vi "Multichannel Recording0.4.vi"() -> ()   [LabVIEW 2014]
uses:
  Enum State Typedef.ctl
  Consumer Data/ Consumer Event Com.ctl
  Data Producer States.ctl
  <vilib>/_DAQmxBase/Internals/DAQmxBase Read (Analog 2D DBL NChan NSamp).vi
  <vilib>/_DAQmxBase/Internals/DAQmxBase Create Channel (AI-Voltage-Basic).vi
  <vilib>/_DAQmxBase/Internals/DAQmxBase Timing (Sample Clock).vi
panel:
  out "Read Data":i32
  out "Data Producer State":T1=enum."Default"
  out "Data Consumer State":T2=enum."Default"
  in  "Open Button":bool
  in  "Tab Control":T3(tab)
  in  "Amplifier Channel 0":T4 {"Amplifier Model" items=["Select a Model", "AM 1700", "BMA 200"]}
  out "Channel 0 Chart":waveform(dbl)(graph)
  in  "User Data Channel 0":T5
  in  "Use Channel 0":bool caption="In Use?"
  out "Channel 1 Chart":waveform(dbl)(graph)
  in  "User Data Channel 1":T5
  in  "Amplifier Channel 1":T4 {"Amplifier Model" items=["Select a Model", "AM 1700", "BMA 200"]}
  in  "Use Channel 1":bool caption="In Use?"
  out "Channel 2 Chart":waveform(dbl)(graph)
  in  "User Data Channel 2":T5
  in  "Amplifier Channel 2":T4 {"Amplifier Model" items=["Select a Model", "AM 1700", "BMA 200"]}
  in  "Use Channel 2":bool caption="In Use?"
  out "Channel 3 Chart":waveform(dbl)(graph)
  in  "User Data Channel 3":T5
  in  "Amplifier Channel 3":T4 {"Amplifier Model" items=["Select a Model", "AM 1700", "BMA 200"]}
  in  "Use Channel 3":bool caption="In Use?"
  out "Overview Chart":waveform(dbl)[](graph)
  in  "Stop Preview":bool
  in  "OK Button":bool
  out "Event State":T6
  in  "Clear Display":bool
  in  "Preview Button":bool
  out "Iterations Recorded":i32
  in  "Recording Time (seconds)":dbl
  in  "Sample Rate":i32=1000
  in  "Stop Button":bool
  out "Start Time hr/min":string
  out "Date mm/dd/yy":string
  in  "Exit Button":bool
  in  "Record Button":bool
  # "MSU EFISH Lab Multi-Channel Electronic Pulse Recorder"
  # "Must enter numbers into here before you start"
  # "Blue for On\nOrange for Off"
  # "DC"
  # "AC"
  # "Blue for AC and Orange for DC"
  # "Blue for On\nOrange for Off"
  # "DC"
  # "AC"
  # "Blue for AC and Orange for DC"
  # "Blue for On\nOrange for Off"
  # "DC"
  # "AC"
  # "Blue for AC and Orange for DC"
  # "Blue for On\nOrange for Off"
  # "DC"
  # "AC"
  # "Blue for AC and Orange for DC"
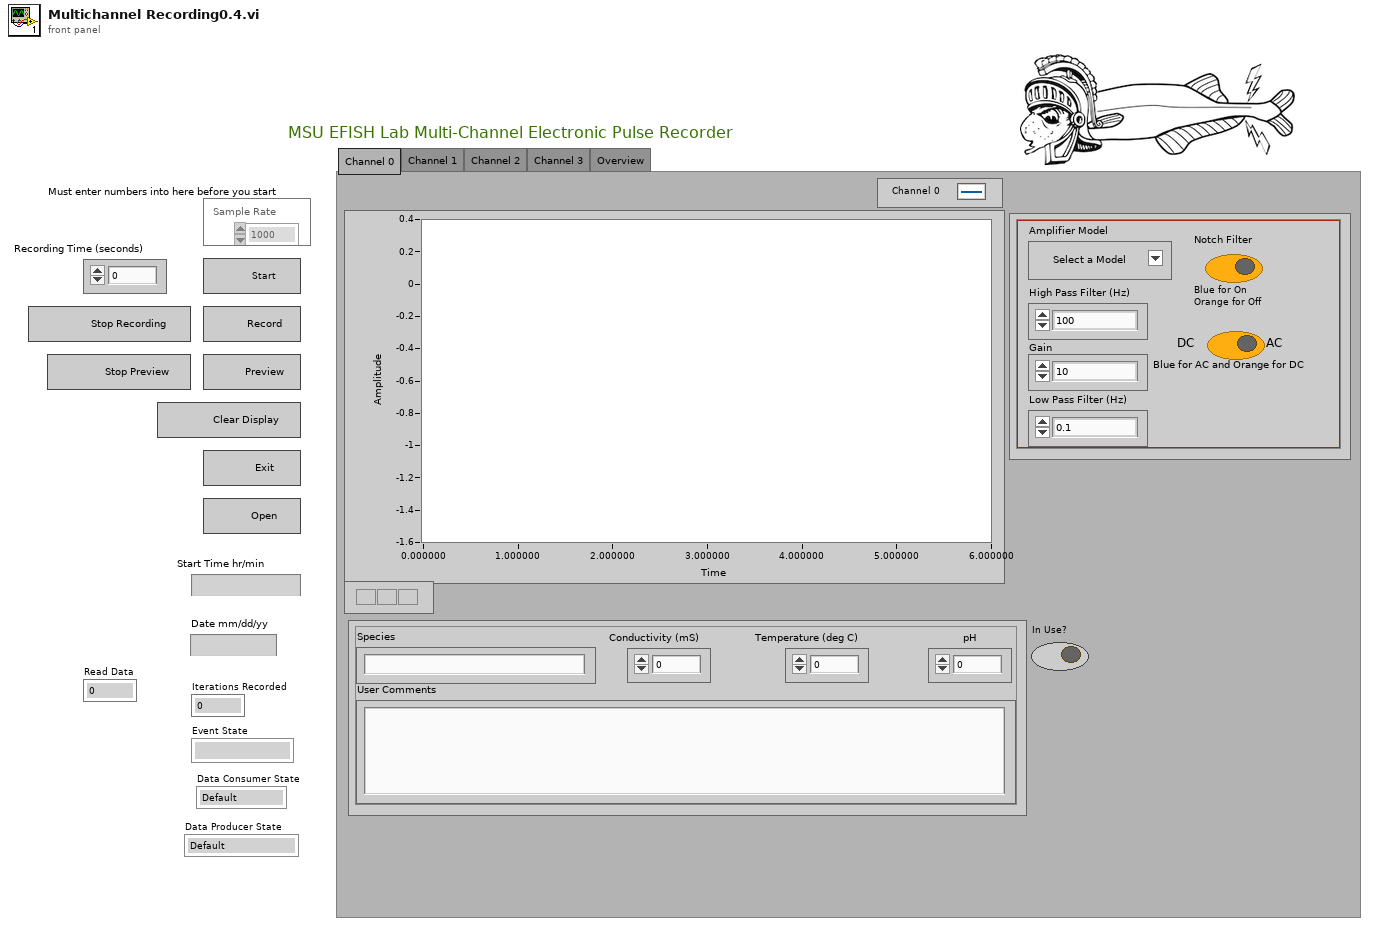
[diagram p1: front panel]
types:
  T1 = typedef "Data Producer States.ctl" = enum16{"Read Data", "Set Sample Clock", "Default", "Exit", "Preview"}
  T2 = typedef "Consumer Data/ Consumer Event Com.ctl" = enum16{"Recording", "Create File", "Clear Memory", "Default", "End File", "Exit", "Set Sample Clock", "Preview"}
  T3 = enum32{"Channel 0", "Channel 1", "Channel 2", "Channel 3", "Overview"}
  T4 = cluster{"Low Pass Filter (Hz)":enum16{"0.1", "1", "3", "10", "30", "100", "300"}, "Gain ":enum16{"10", "20", "50", "100", "200", "500", "1000", "2k", "5k", "10k", "20k", "50k"}, "High Pass Filter (Hz)":enum16{"100", "500", "1000", "3000", "5000", "10,000", "20,000", "30,000", "50,000"}, "Notch Filter":bool, "Amplifier Model":u16, "AC/DC Switch":bool}
  T5 = cluster{"pH":dbl, "Conductivity (mS)":dbl, "Temperature (deg C)":dbl, "User Comments":string, "Species":string}
  T6 = typedef "Enum State Typedef.ctl" = enum16{"", "Open FIle", "Beginning State", "Set the Sample Clock", "Prepreview Handling", "Clear Display", "Preview Data", "Stop", "Exit", "Record", "Create File"}
  T7 = enum8{"Enabled", "Disabled", "Disabled and Grayed Out"}
  T8 = enum16{"Recording", "Create File", "Clear Memory", "Default"}
  T9 = cluster{"Refnum out":refnum<k34>, "Refnum out":refnum<k34>, "Refnum out":refnum<k34>, "Refnum out":refnum<k34>}
  T10 = cluster{"Use Channel 0":bool, "Use Channel 1":bool, "Use Channel 2":bool, "Use Channel 3":bool}
  T11 = cluster{"tdms file out":refnum<k34>, "tdms file out":refnum<k34>, "tdms file out":refnum<k34>, "tdms file out":refnum<k34>}
  T12 = cluster{"Waveform":waveform(dbl), "Waveform":waveform(dbl), "Waveform":waveform(dbl), "Waveform":waveform(dbl)}
  T13 = cluster{"Waveform":waveform(dbl), "Waveform":waveform(dbl), "Waveform":waveform(dbl), "Waveform":waveform(dbl), waveform(dbl)[]}
  T14 = enum16{"Read Data", "Set Sample Clock", "Default", "Exit"}
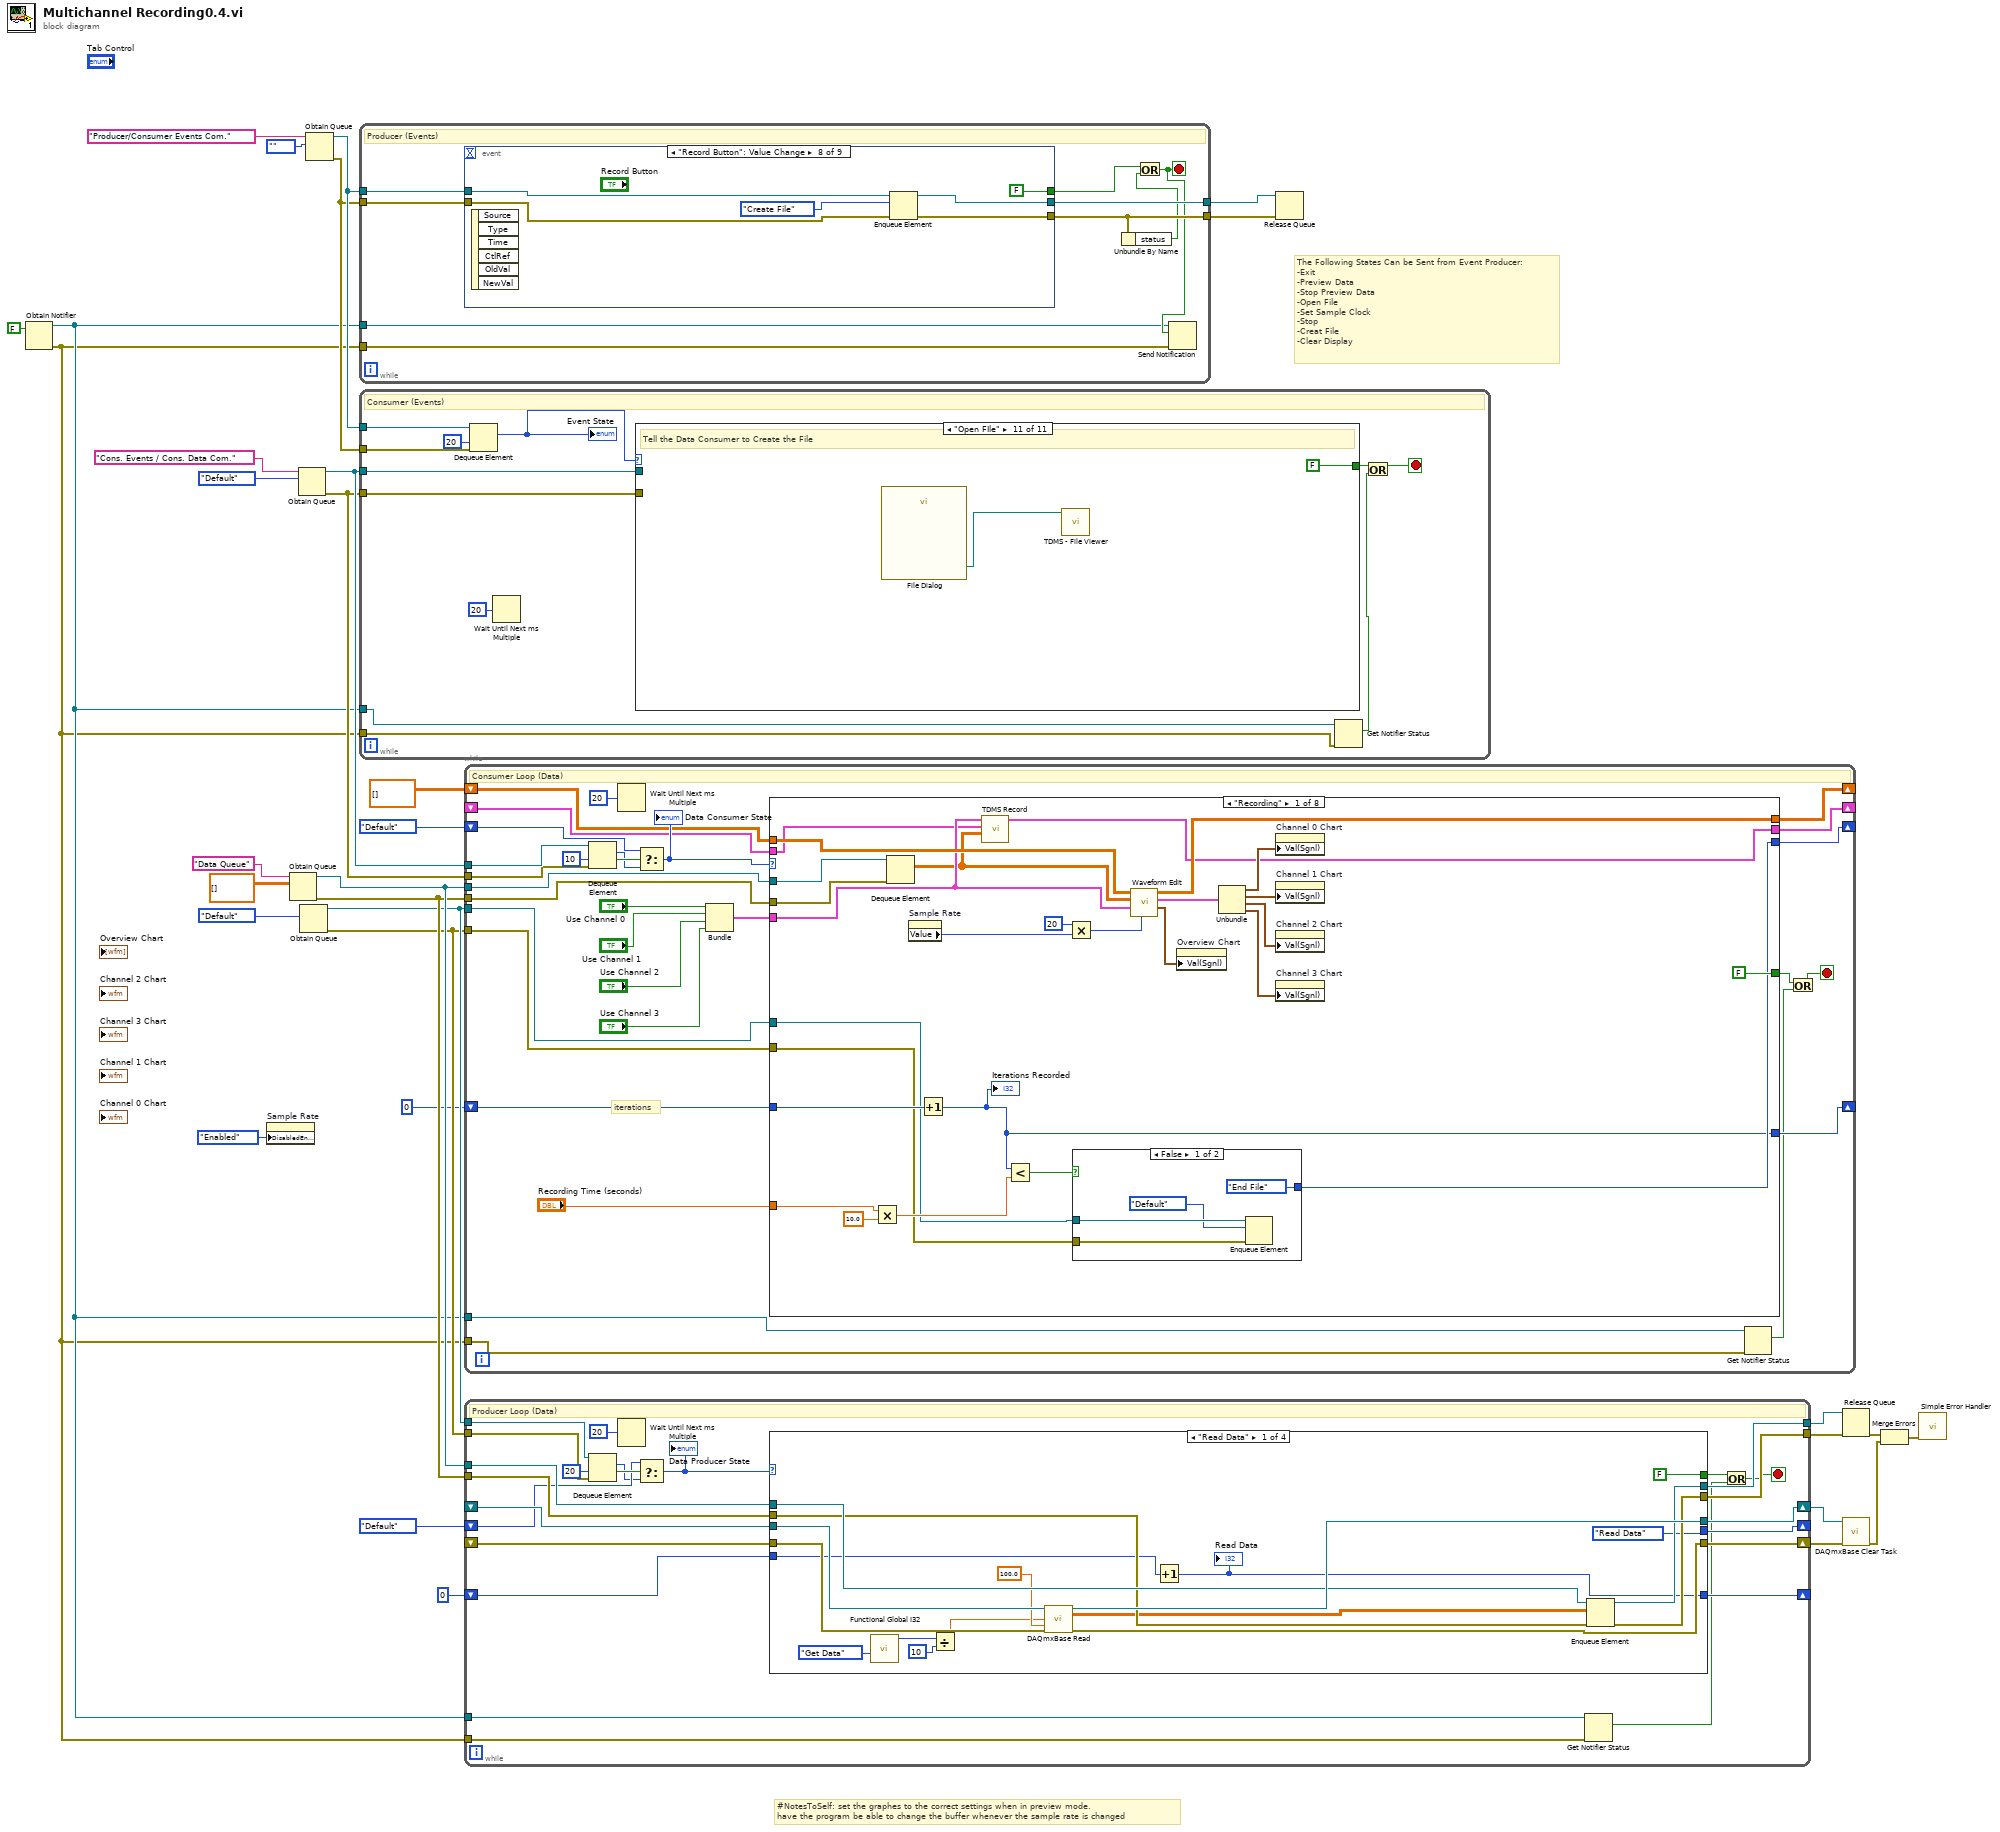
[diagram p0: block diagram]
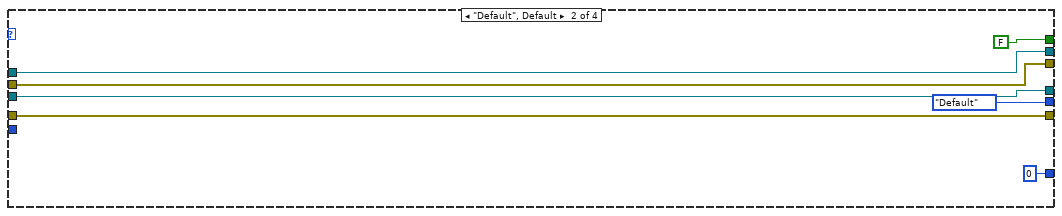
[diagram p2: hidden frame]
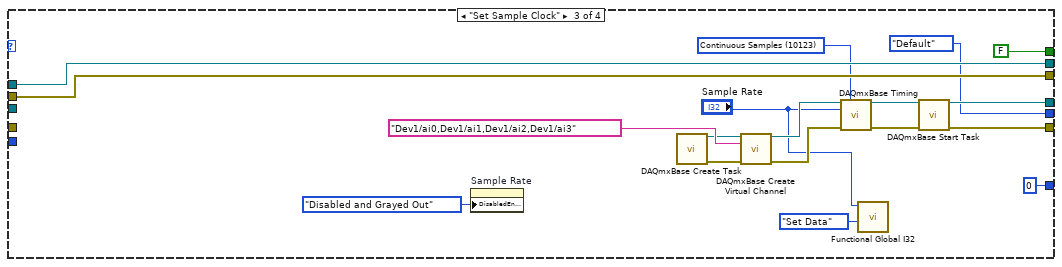
[diagram p3: hidden frame]
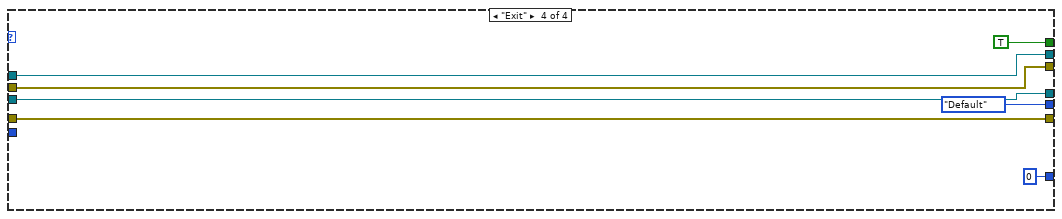
[diagram p4: hidden frame]
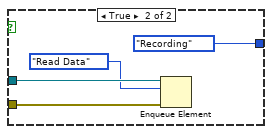
[diagram p5: hidden frame]
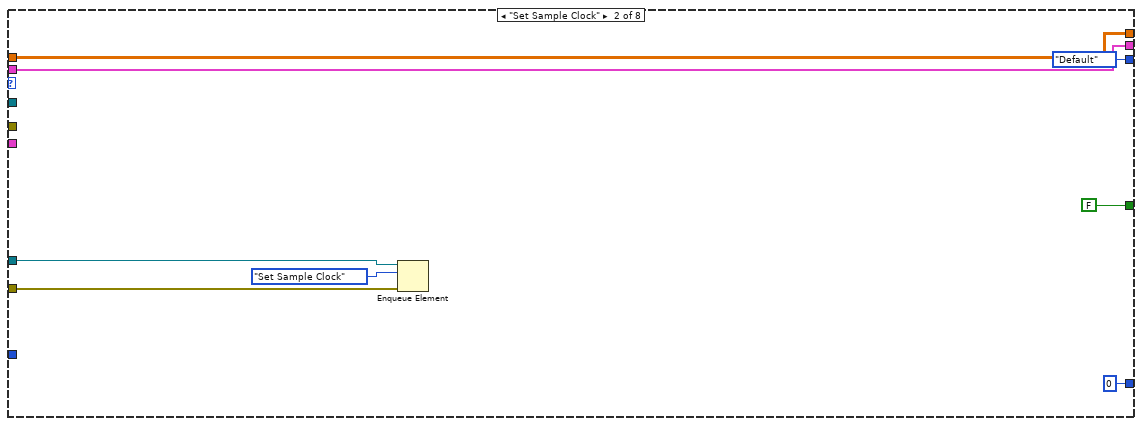
[diagram p6: hidden frame]
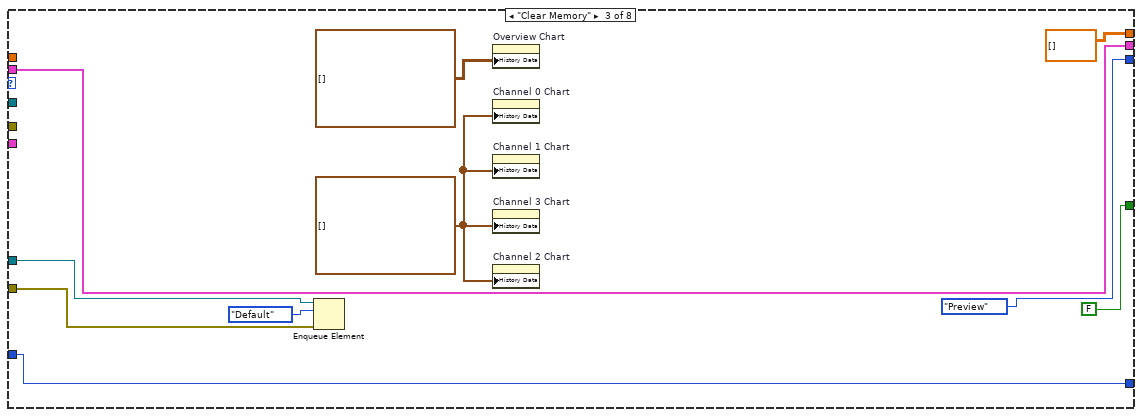
[diagram p7: hidden frame]
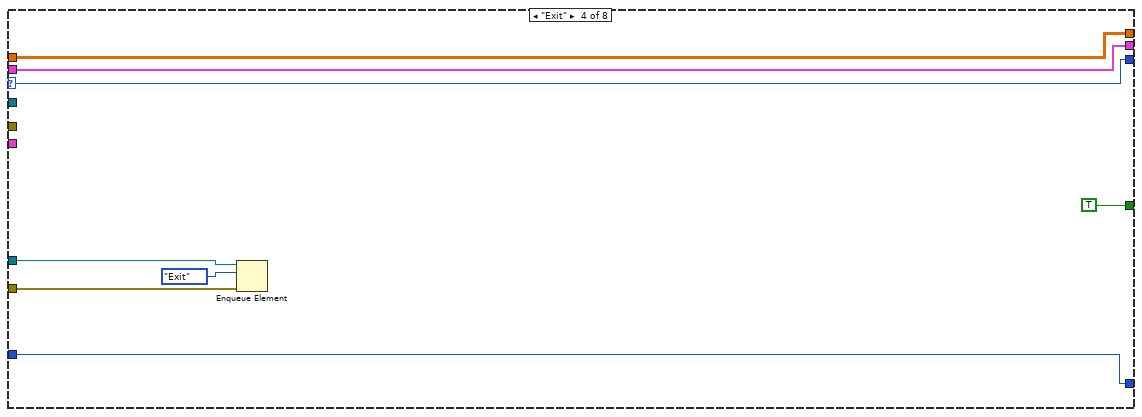
[diagram p8: hidden frame]
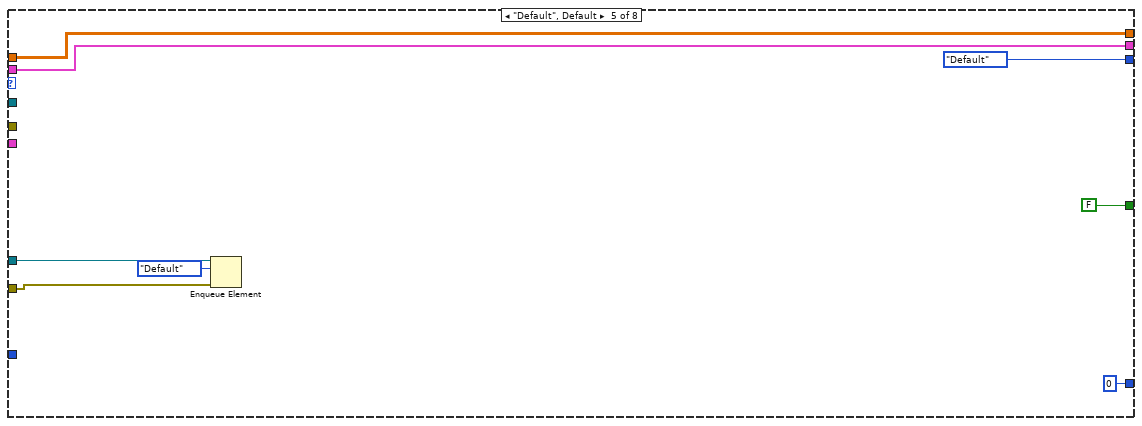
[diagram p9: hidden frame]
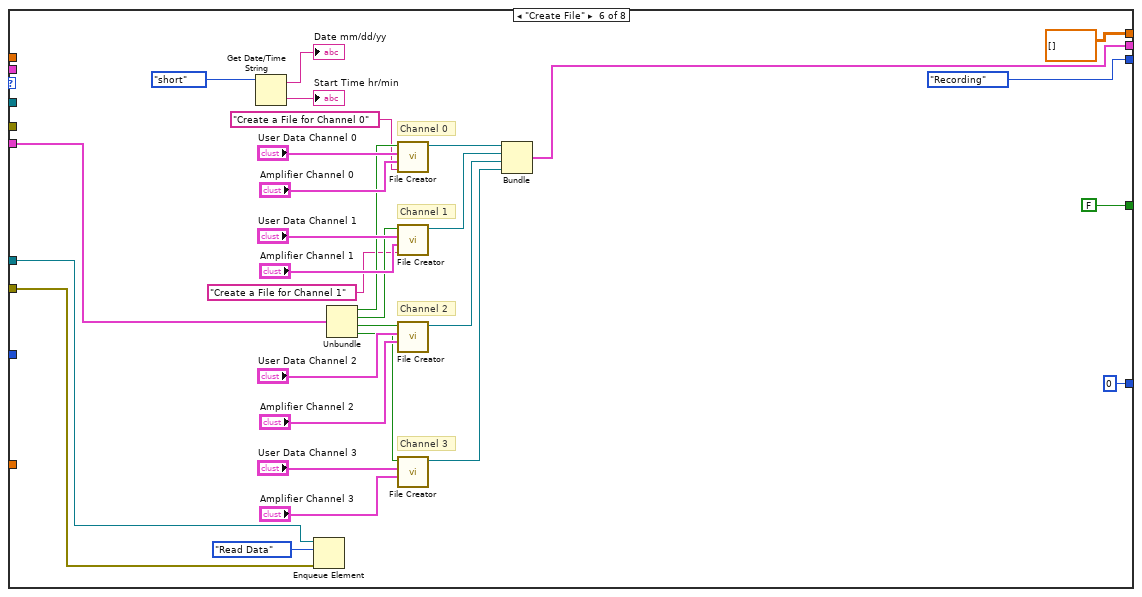
[diagram p10: hidden frame]
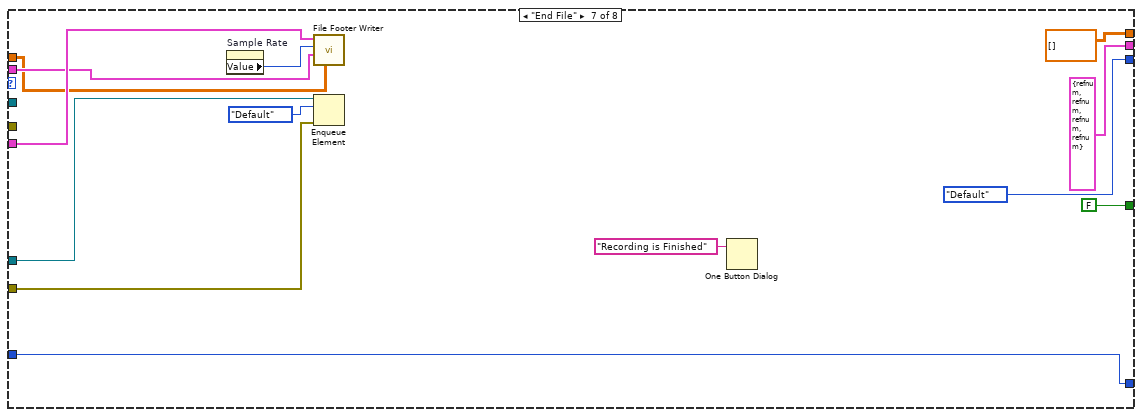
[diagram p11: hidden frame]
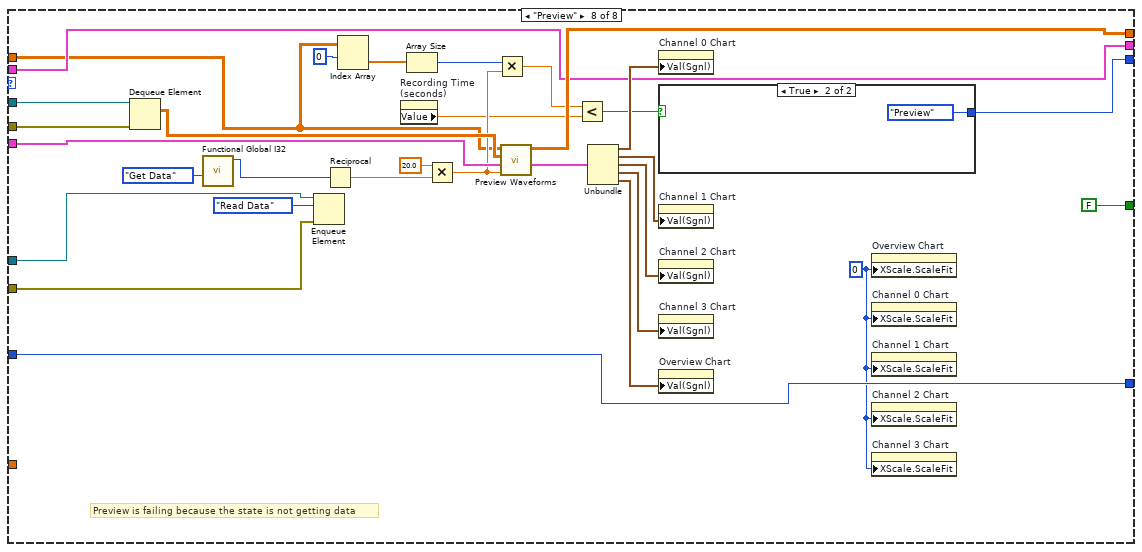
[diagram p12: hidden frame]
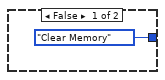
[diagram p13: hidden frame]
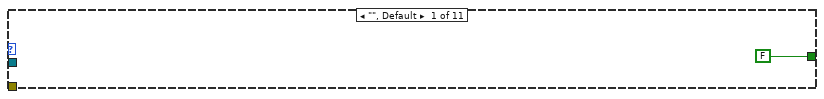
[diagram p14: hidden frame]
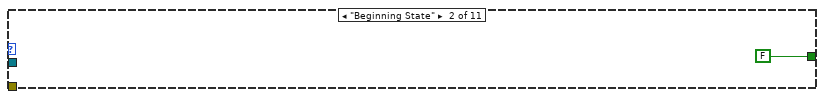
[diagram p15: hidden frame]
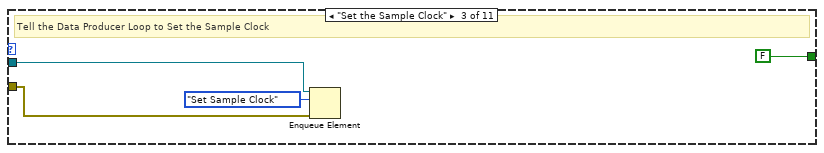
[diagram p16: hidden frame]
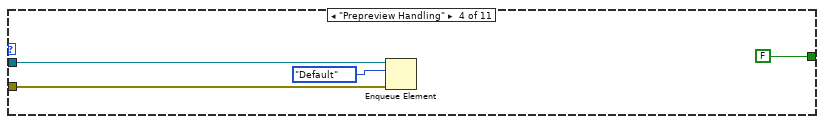
[diagram p17: hidden frame]
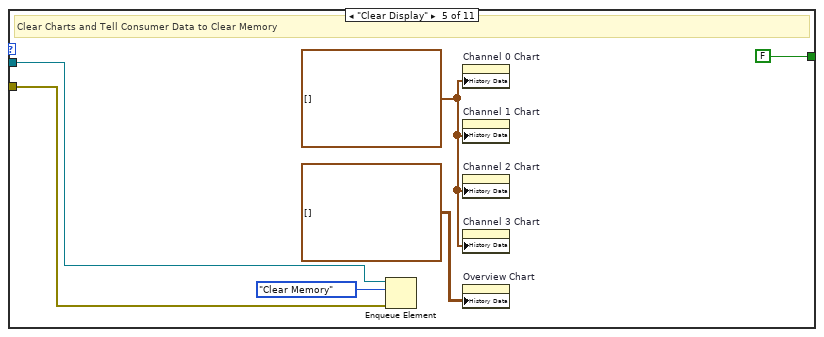
[diagram p18: hidden frame]
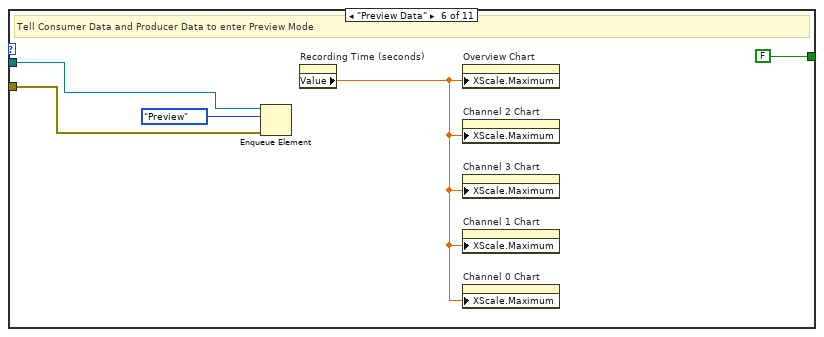
[diagram p19: hidden frame]
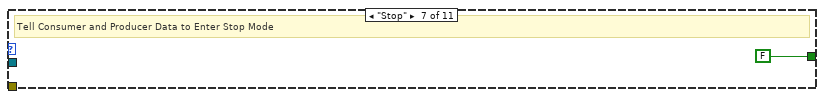
[diagram p20: hidden frame]
diagram:
  # "#NotesToSelf: set the graphes to the correct settings when in preview mode.\nhave the program be able to change the buffer whenever the sample rate is changed"
  # "The Following States Can be Sent from Event Producer:\n-Exit\n-Preview Data\n-Stop Preview Data\n-Open File\n-Set Sample Clock\n-Stop\n-Creat File\n-Clear Display"
  n1 = Obtain Notifier(notification data type=FALSE) -> (notifier out=w2:refnum<notifier>, error out=w1:errorcluster)  [unwired: 3 in, 1 out]
  n2 = property on="Sample Rate" class="DigNum (strict)"("DisabledEnum"=T7."Enabled" ("Disabled")) -> ()  [unwired: 2 in, 2 out]
  n3 = Obtain Queue(name (unnamed)="Data Queue", element data type=dbl[][] []) -> (queue out=w28:refnum<queue>, error out=w27:errorcluster)  [unwired: 3 in, 1 out]
  n4 = Obtain Queue(name (unnamed)="Cons. Events / Cons. Data Com.", element data type=Consumer_Data/_Consumer_Event_Com."Default") -> (queue out=w20:refnum<queue>, error out=w19:errorcluster)  [unwired: 3 in, 1 out]
  n5 = Obtain Queue(element data type=Data_Producer_States."Default") -> (queue out=w9:refnum<queue>, error out=w8:errorcluster)  [unwired: 4 in, 1 out]
  n6 = Obtain Queue(name (unnamed)="Producer/Consumer Events Com.", element data type=Enum_State_Typedef."" ("State")) -> (queue out=w32:refnum<queue>, error out=w31:errorcluster)  [unwired: 3 in, 1 out]
  n7 = while {
    tunnel: w32 -> [w42]
    tunnel: w31 -> [w41]
    tunnel: [w40] -> w26
    tunnel: [w39] -> w25
    tunnel: w2 -> [w35]
    tunnel: w1 -> [w34]
    stop <- w36 stop-if-true
    # "Producer (Events)"
    n8 = event shown="[7] \"Record Button\": Value Change" {
      selector: _ -> [_ _ _ _ _ _ _ _ _]
      dyn-events: _ -> [_ _ _ _ _ _ _ _ _]
      timeout: _ -> [_ _ _ _ _ _ _ _ _]
      tunnel: [FALSE ("Exit Button") "Exit Button" FALSE ("Exit Button") FALSE ("Exit Button") FALSE ("Exit Button") FALSE ("Exit Button") FALSE ("Exit Button") FALSE ("Exit Button") FALSE ("Exit Button")] -> w38
      tunnel: w42 -> [w44 w50 w57 w63 w69 w75 w81 w87 w93]
      tunnel: w41 -> [w43 w49 w56 w62 w68 w74 w80 w86 w92]
      tunnel: [w44 w47 w53 w59 w65 w71 w77 w83 w89] -> w40
      tunnel: [w43 w46 w52 w58 w64 w70 w76 w82 w88] -> w39
      event Timeout {
        n9 = event-data() -> ()  [unwired: 1 in, 3 out]
      }
      event "Exit Button": Value Change {
        n10 = event-data() -> ()  [unwired: 1 in, 1 out]
        n11 = Enqueue Element(queue=w50, element=Enum_State_Typedef."Exit", error in (no error)=w49) -> (queue out=w47:refnum<queue>, error out=w46:errorcluster)  [unwired: 1 in, 1 out]
      }
      event "Preview Button": Value Change {
        n12 = event-data() -> ()  [unwired: 1 in, 6 out]
        n13 = Enqueue Element(queue=w57, element=Enum_State_Typedef."Preview Data", error in (no error)=w56) -> (queue out=w53:refnum<queue>, error out=w52:errorcluster)  [unwired: 1 in, 1 out]
      }
      event "Stop Preview": Value Change {
        n14 = event-data() -> ()  [unwired: 1 in, 6 out]
        n15 = Enqueue Element(queue=w63, element=Enum_State_Typedef."Prepreview Handling", error in (no error)=w62) -> (queue out=w59:refnum<queue>, error out=w58:errorcluster)  [unwired: 1 in, 1 out]
      }
      event "Open Button": Value Change {
        n16 = event-data() -> ()  [unwired: 1 in, 6 out]
        n17 = Enqueue Element(queue=w69, element=Enum_State_Typedef."Open FIle", error in (no error)=w68) -> (queue out=w65:refnum<queue>, error out=w64:errorcluster)  [unwired: 1 in, 1 out]
      }
      event "OK Button": Value Change {
        n18 = event-data() -> ()  [unwired: 1 in, 6 out]
        n19 = Enqueue Element(queue=w75, element=Enum_State_Typedef."Set the Sample Clock", error in (no error)=w74) -> (queue out=w71:refnum<queue>, error out=w70:errorcluster)  [unwired: 1 in, 1 out]
      }
      event "Stop Button": Value Change {
        n20 = event-data() -> ()  [unwired: 1 in, 6 out]
        n21 = Enqueue Element(queue=w81, element=Enum_State_Typedef."Stop", error in (no error)=w80) -> (queue out=w77:refnum<queue>, error out=w76:errorcluster)  [unwired: 1 in, 1 out]
      }
      event "Record Button": Value Change {
        n22 = event-data() -> ()  [unwired: 1 in, 6 out]
        n23 = Enqueue Element(queue=w87, element=Enum_State_Typedef."Create File", error in (no error)=w86) -> (queue out=w83:refnum<queue>, error out=w82:errorcluster)  [unwired: 1 in, 1 out]
      }
      event "Clear Display": Value Change {
        n24 = event-data() -> ()  [unwired: 1 in, 6 out]
        n25 = Enqueue Element(queue=w93, element=Enum_State_Typedef."Clear Display", error in (no error)=w92) -> (queue out=w89:refnum<queue>, error out=w88:errorcluster)  [unwired: 1 in, 1 out]
      }
    }
    n26 = Unbundle By Name(w39) -> ("status"=w37:bool)
    n27 = Or(x=w38, y=w37) -> (x .or. y?=w36:bool)
    n28 = Send Notification(notification=w36, notifier=w35, error in (no error)=w34) -> ()  [unwired: 2 out]
  }
  n29 = while {
    tunnel: w32 -> [w105]
    tunnel: w31 -> [w104]
    tunnel: w20 -> [w103]
    tunnel: w19 -> [w102]
    tunnel: w2 -> [w97]
    tunnel: w1 -> [w96]
    stop <- w95 stop-if-true
    # "Consumer (Events)"
    n30 = Dequeue Element(queue=w105, timeout in ms (-1)=20, error in (no error)=w104) -> (element=w100:T6)  [unwired: 3 out]
    "Event State" <- w100
    n31 = Wait Until Next ms Multiple(millisecond multiple=u32 20) -> ()  [unwired: 1 out]
    n32 = case shown="\"Open FIle\"" w100 {
      tunnel: w103 -> [_ _ w110 w114 w118 w124 _ w131 _ w136 _]
      tunnel: w102 -> [_ _ w109 w113 w117 w123 _ w130 _ w135 _]
      tunnel: [FALSE FALSE FALSE FALSE FALSE FALSE FALSE TRUE FALSE FALSE FALSE] -> w101
      frame "", Default {
      }
      frame "Beginning State" {
      }
      frame "Set the Sample Clock" {
        # "Tell the Data Producer Loop to Set the Sample Clock"
        n33 = Enqueue Element(queue=w110, element=Consumer_Data/_Consumer_Event_Com."Set Sample Clock", error in (no error)=w109) -> ()  [unwired: 1 in, 3 out]
      }
      frame "Prepreview Handling" {
        n34 = Enqueue Element(queue=w114, element=Consumer_Data/_Consumer_Event_Com."Default", error in (no error)=w113) -> ()  [unwired: 1 in, 3 out]
      }
      frame "Clear Display" {
        w120 = waveform(dbl)[] [] ("History Data")
        # "Clear Charts and Tell Consumer Data to Clear Memory"
        n35 = Enqueue Element(queue=w118, element=Consumer_Data/_Consumer_Event_Com."Clear Memory", error in (no error)=w117) -> ()  [unwired: 1 in, 3 out]
        n36 = property on="Channel 0 Chart" class="WFChart (strict)"("History Data"=w120) -> ()  [unwired: 2 in, 2 out]
        n37 = property on="Channel 1 Chart" class="WFChart (strict)"("History Data"=w120) -> ()  [unwired: 2 in, 2 out]
        n38 = property on="Channel 2 Chart" class="WFChart (strict)"("History Data"=w120) -> ()  [unwired: 2 in, 2 out]
        n39 = property on="Channel 3 Chart" class="WFChart (strict)"("History Data"=w120) -> ()  [unwired: 2 in, 2 out]
        n40 = property on="Overview Chart" class="WFChart (strict)"("History Data"=waveform(dbl)[][] []) -> ()  [unwired: 2 in, 2 out]
      }
      frame "Preview Data" {
        # "Tell Consumer Data and Producer Data to enter Preview Mode"
        n41 = Enqueue Element(queue=w124, element=Consumer_Data/_Consumer_Event_Com."Preview", error in (no error)=w123) -> ()  [unwired: 1 in, 3 out]
        n42 = property on="Recording Time (seconds)" class="DigNum (strict)"() -> ("Value"=w125:dbl)  [unwired: 2 in, 2 out]
        n43 = property on="Overview Chart" class="WFChart (strict)"("XScale.Maximum"=w125) -> ()  [unwired: 2 in, 2 out]
        n44 = property on="Channel 2 Chart" class="WFChart (strict)"("XScale.Maximum"=w125) -> ()  [unwired: 2 in, 2 out]
        n45 = property on="Channel 3 Chart" class="WFChart (strict)"("XScale.Maximum"=w125) -> ()  [unwired: 2 in, 2 out]
        n46 = property on="Channel 1 Chart" class="WFChart (strict)"("XScale.Maximum"=w125) -> ()  [unwired: 2 in, 2 out]
        n47 = property on="Channel 0 Chart" class="WFChart (strict)"("XScale.Maximum"=w125) -> ()  [unwired: 2 in, 2 out]
      }
      frame "Stop" {
        # "Tell Consumer and Producer Data to Enter Stop Mode"
      }
      frame "Exit" {
        # "Tell Producer and Consumer Data to end themselves then End the Program"
        n48 = Enqueue Element(queue=w131, element=Consumer_Data/_Consumer_Event_Com."Exit", error in (no error)=w130) -> ()  [unwired: 1 in, 3 out]
      }
      frame "Record" {
        # "(I dont think that this case will exist)"
      }
      frame "Create File" {
        w133 = u8 2 ("X Scale.Scale Fit")
        # "Let Consumer Data Create File"
        n49 = Enqueue Element(queue=w136, element=Consumer_Data/_Consumer_Event_Com."Create File", error in (no error)=w135) -> ()  [unwired: 1 in, 3 out]
        n50 = property on="Overview Chart" class="WFChart (strict)"("XScale.ScaleFit"=w133) -> ()  [unwired: 2 in, 2 out]
        n51 = property on="Channel 3 Chart" class="WFChart (strict)"("XScale.ScaleFit"=w133) -> ()  [unwired: 2 in, 2 out]
        n52 = property on="Channel 2 Chart" class="WFChart (strict)"("XScale.ScaleFit"=w133) -> ()  [unwired: 2 in, 2 out]
        n53 = property on="Channel 1 Chart" class="WFChart (strict)"("XScale.ScaleFit"=w133) -> ()  [unwired: 2 in, 2 out]
        n54 = property on="Channel 0 Chart" class="WFChart (strict)"("XScale.ScaleFit"=w133) -> ()  [unwired: 2 in, 2 out]
      }
      frame "Open FIle" {
        # "Tell the Data Consumer to Create the File"
        n55 = call "File Dialog"() -> ("selected path"=w138:path)  [unwired: 12 in, 3 out]
        n56 = call <vilib>:"TDMS - File Viewer.vi"("file path"=w138) -> ()  [unwired: 5 in, 2 out]
      }
    }
    n57 = Get Notifier Status(notifier=w97, error in (no error)=w96) -> (current notification=w94:bool)  [unwired: 4 out]
    n58 = Or(x=w101, y=w94) -> (x .or. y?=w95:bool)
  }
  n59 = while {
    tunnel: w28 -> [w162]
    tunnel: w27 -> [w161]
    tunnel: w20 -> [w169]
    tunnel: w19 -> [w168]
    shift-right: [w163] -> _
    shift-left: Consumer_Data/_Consumer_Event_Com."Default" -> [w164]
    shift-right: [w157] -> _
    shift-left: dbl[][] [] -> [w160]
    shift-right: [w156] -> _
    shift-left: _ -> [w155]
    tunnel: w9 -> [w153]
    tunnel: w8 -> [w152]
    shift-right: [w148] -> _
    shift-left: 0 -> [w150]
    tunnel: w2 -> [w142]
    tunnel: w1 -> [w141]
    stop <- w144 stop-if-true
    # "iterations"
    # "Consumer Loop (Data)"
    n60 = Dequeue Element(queue=w169, timeout in ms (-1)=10, error in (no error)=w168) -> (element=w166:T2, timed out?=w167:bool)  [unwired: 2 out]
    n61 = Wait Until Next ms Multiple(millisecond multiple=u32 20) -> ()  [unwired: 1 out]
    n62 = Select(t=w164, s=w167, f=w166) -> (s? t:f=w165:T2)
    "Data Consumer State" <- w165
    n63 = Bundle("Use Channel 0"="Use Channel 0", "Use Channel 1"="Use Channel 1", "Use Channel 2"="Use Channel 2", "Use Channel 3"="Use Channel 3") -> (w158:T10)  [unwired: 1 in]
    n64 = case shown="\"Recording\"" w165 {
      selector: w165 -> [_ _ _ w228 _ _ _ _]
      tunnel: [w174 Consumer_Data/_Consumer_Event_Com."Default" Consumer_Data/_Consumer_Event_Com."Preview" w228 T8."Default" Consumer_Data/_Consumer_Event_Com."Recording" Consumer_Data/_Consumer_Event_Com."Default" w290] -> w163
      tunnel: w162 -> [w195 _ _ _ _ _ _ w312]
      tunnel: w161 -> [w194 _ _ _ _ _ _ w311]
      tunnel: [FALSE FALSE FALSE TRUE FALSE FALSE FALSE FALSE] -> w143
      tunnel: w160 -> [w193 w209 _ w229 w236 _ w279 w297]
      tunnel: w158 -> [w182 _ _ _ _ w262 w281 w309]
      tunnel: [w183 w209 dbl[][] [] ("Output Decimated Data") w229 w236 dbl[][] [] ("Output Decimated Data") dbl[][] [] ("Output Data") w306] -> w157
      tunnel: [w180 w208 w219 w227 w235 w245 T9 {"Refnum out"=refnum, "Refnum out"=refnum, "Refnum out"=refnum, "Refnum out"=refnum} ("Output TDMS File Cluster") w299] -> w156
      tunnel: w155 -> [w170 w208 w219 w227 w235 _ w280 w299]
      tunnel: w153 -> [w173 w212 w216 w226 w233 w244 w273 w288]
      tunnel: w152 -> [w172 w211 w215 w225 w232 w243 w272 w287]
      tunnel: w150 -> [w179 _ w213 w223 _ _ w270 w285]
      tunnel: "Recording Time (seconds)" -> [w178 _ _ _ _ _ _ _]
      tunnel: [w171 0 w213 w223 0 0 w270 w285] -> w148
      frame "Recording" {
        n65 = Multiply(x=w178, y=10.0) -> (x*y=w176:dbl)
        n66 = Dequeue Element(queue=w195, error in (no error)=w194) -> (element=w181:dbl[][])  [unwired: 1 in, 3 out]
        n67 = property on="Sample Rate" class="DigNum (strict)"() -> ("Value"=w192:i32)  [unwired: 2 in, 2 out]
        n68 = Increment(x=w179) -> (x+1=w171:i32)
        "Iterations Recorded" <- w171
        n69 = call "TDMS Record.vi"("Data"=w181, "Input TDMS File Cluster"=w170, "In Use Cluster"=w182) -> ("Output TDMS File Cluster"=w180:T11)  [unwired: 8 in]
        n70 = Less?(x=w171, y=w176) -> (x < y?=w175:bool)
        n71 = Multiply(x=20, y=w192) -> (x*y=w190:i32)
        n72 = case shown="False" w175 {
          tunnel: [Consumer_Data/_Consumer_Event_Com."End File" Consumer_Data/_Consumer_Event_Com."Recording"] -> w174
          tunnel: w173 -> [w199 w203]
          tunnel: w172 -> [w198 w202]
          frame False {
            n73 = Enqueue Element(queue=w199, element=Data_Producer_States."Default", error in (no error)=w198) -> ()  [unwired: 1 in, 3 out]
          }
          frame True {
            n74 = Enqueue Element(queue=w203, element=Data_Producer_States."Read Data", error in (no error)=w202) -> ()  [unwired: 1 in, 3 out]
          }
        }
        n75 = call "Waveform Edit.vi"("Change in Time"=w190, "In Use Cluster"=w182, "New Data"=w181, "Old Data"=w193) -> ("Overview Chart Data"=w184:waveform(dbl)[], "Output Waveform Cluster"=w189:T12, "Output Decimated Data"=w183:dbl[][])  [unwired: 5 in]
        n76 = property on="Overview Chart" class="WFChart (strict)"("Val(Sgnl)"=w184) -> ()  [unwired: 2 in, 2 out]
        n77 = Unbundle(w189) -> ("Waveform"=w188:waveform(dbl), "Waveform"=w187:waveform(dbl), "Waveform"=w186:waveform(dbl), "Waveform"=w185:waveform(dbl))
        n78 = property on="Channel 0 Chart" class="WFChart (strict)"("Val(Sgnl)"=w188) -> ()  [unwired: 2 in, 2 out]
        n79 = property on="Channel 1 Chart" class="WFChart (strict)"("Val(Sgnl)"=w187) -> ()  [unwired: 2 in, 2 out]
        n80 = property on="Channel 2 Chart" class="WFChart (strict)"("Val(Sgnl)"=w186) -> ()  [unwired: 2 in, 2 out]
        n81 = property on="Channel 3 Chart" class="WFChart (strict)"("Val(Sgnl)"=w185) -> ()  [unwired: 2 in, 2 out]
      }
      frame "Set Sample Clock" {
        n82 = Enqueue Element(queue=w212, element=Data_Producer_States."Set Sample Clock", error in (no error)=w211) -> ()  [unwired: 1 in, 3 out]
      }
      frame "Clear Memory" {
        w217 = waveform(dbl)[] [] ("History Data")
        n83 = Enqueue Element(queue=w216, element=Data_Producer_States."Default", error in (no error)=w215) -> ()  [unwired: 1 in, 3 out]
        n84 = property on="Overview Chart" class="WFChart (strict)"("History Data"=waveform(dbl)[][] []) -> ()  [unwired: 2 in, 2 out]
        n85 = property on="Channel 0 Chart" class="WFChart (strict)"("History Data"=w217) -> ()  [unwired: 2 in, 2 out]
        n86 = property on="Channel 1 Chart" class="WFChart (strict)"("History Data"=w217) -> ()  [unwired: 2 in, 2 out]
        n87 = property on="Channel 3 Chart" class="WFChart (strict)"("History Data"=w217) -> ()  [unwired: 2 in, 2 out]
        n88 = property on="Channel 2 Chart" class="WFChart (strict)"("History Data"=w217) -> ()  [unwired: 2 in, 2 out]
      }
      frame "Exit" {
        n89 = Enqueue Element(queue=w226, element=Data_Producer_States."Exit", error in (no error)=w225) -> ()  [unwired: 1 in, 3 out]
      }
      frame "Default", Default {
        n90 = Enqueue Element(queue=w233, element=Data_Producer_States."Default", error in (no error)=w232) -> ()  [unwired: 1 in, 3 out]
      }
      frame "Create File" {
        # "Channel 3"
        # "Channel 2"
        # "Channel 1"
        # "Channel 0"
        n91 = Get Date/Time String(date format (0)=enum16{"short", "long", "abbreviated"}."short") -> (date string=→"Date mm/dd/yy":string, time string=→"Start Time hr/min":string)  [unwired: 2 in]
        n92 = Enqueue Element(queue=w244, element=Data_Producer_States."Read Data", error in (no error)=w243) -> ()  [unwired: 1 in, 3 out]
        n93 = Unbundle(w262) -> ("Use Channel 0"=w255:bool, "Use Channel 1"=w254:bool, "Use Channel 2"=w253:bool, "Use Channel 3"=w252:bool)
        n94 = call "File Creator.vi"("prompt"="Create a File for Channel 0", "Amplifier Channel 1"="Amplifier Channel 0", "User Data Channel 1"="User Data Channel 0", "Use Channel in"=w255) -> ("Refnum out"=w251:refnum<k34>)  [unwired: 7 in]
        n95 = call "File Creator.vi"("prompt"="Create a File for Channel 1", "Amplifier Channel 1"="Amplifier Channel 1", "User Data Channel 1"="User Data Channel 1", "Use Channel in"=w254) -> ("Refnum out"=w250:refnum<k34>)  [unwired: 7 in]
        n96 = call "File Creator.vi"("Amplifier Channel 1"="Amplifier Channel 2", "User Data Channel 1"="User Data Channel 2", "Use Channel in"=w253) -> ("Refnum out"=w249:refnum<k34>)  [unwired: 8 in]
        n97 = call "File Creator.vi"("Amplifier Channel 1"="Amplifier Channel 3", "User Data Channel 1"="User Data Channel 3", "Use Channel in"=w252) -> ("Refnum out"=w248:refnum<k34>)  [unwired: 8 in]
        n98 = Bundle("Refnum out"=w251, "Refnum out"=w250, "Refnum out"=w249, "Refnum out"=w248) -> (w245:T9)  [unwired: 1 in]
      }
      frame "End File" {
        n99 = property on="Sample Rate" class="DigNum (strict)"() -> ("Value"=w278:i32)  [unwired: 2 in, 2 out]
        n100 = call "File Footer Writer.vi"("Old Data"=w279, "TDMS File Cluster"=w280, "Sample Rate"=w278, "In Use Cluster"=w281) -> ()  [unwired: 8 in]
        n101 = Enqueue Element(queue=w273, element=Data_Producer_States."Default", error in (no error)=w272) -> ()  [unwired: 1 in, 3 out]
        n102 = One Button Dialog(message="Recording is Finished") -> ()  [unwired: 1 in, 1 out]
      }
      frame "Preview" {
        w282 = u8 0 ("X Scale.Scale Fit")
        # "Preview is failing because the state is not getting data"
        n103 = Dequeue Element(queue=w312, error in (no error)=w311) -> (element=w310:dbl[][])  [unwired: 1 in, 3 out]
        n104 = call "Functional Global I32.vi"("Enum"=enum16{"Set Data", "Get Data"}."Get Data") -> ("Integer"=w283:i32)  [unwired: 10 in]
        n105 = Enqueue Element(queue=w288, element=Data_Producer_States."Read Data", error in (no error)=w287) -> ()  [unwired: 1 in, 3 out]
        n106 = Reciprocal(x=w283) -> (1/x=w308:dbl)
        n107 = Index Array(array=w297, index (row)=0) -> (element=w295:dbl[])  [unwired: 1 in]
        n108 = property on="Recording Time (seconds)" class="DigNum (strict)"() -> ("Value"=w292:dbl)  [unwired: 2 in, 2 out]
        n109 = Array Size(array=w295) -> (size(s)=w294:i32)
        n110 = Multiply(x=20.0, y=w308) -> (x*y=w298:dbl)
        n111 = Multiply(x=w294, y=w298) -> (x*y=w293:dbl)
        n112 = call "Preview Waveforms.vi"("Change in Time"=w298, "In Use Cluster"=w309, "Input Read Data"=w310, "Input Decimated Data"=w297) -> ("Output Waveform Cluster"=w305:T13, "Output Data"=w306:dbl[][])  [unwired: 6 in]
        n113 = Less?(x=w293, y=w292) -> (x < y?=w291:bool)
        n114 = Unbundle(w305) -> ("Waveform"=w304:waveform(dbl), "Waveform"=w303:waveform(dbl), "Waveform"=w302:waveform(dbl), "Waveform"=w301:waveform(dbl), w300:waveform(dbl)[])
        n115 = property on="Channel 0 Chart" class="WFChart (strict)"("Val(Sgnl)"=w304) -> ()  [unwired: 2 in, 2 out]
        n116 = case shown="True" w291 {
          tunnel: [Consumer_Data/_Consumer_Event_Com."Clear Memory" Consumer_Data/_Consumer_Event_Com."Preview"] -> w290
          frame False {
          }
          frame True {
          }
        }
        n117 = property on="Channel 1 Chart" class="WFChart (strict)"("Val(Sgnl)"=w303) -> ()  [unwired: 2 in, 2 out]
        n118 = property on="Channel 2 Chart" class="WFChart (strict)"("Val(Sgnl)"=w302) -> ()  [unwired: 2 in, 2 out]
        n119 = property on="Channel 3 Chart" class="WFChart (strict)"("Val(Sgnl)"=w301) -> ()  [unwired: 2 in, 2 out]
        n120 = property on="Overview Chart" class="WFChart (strict)"("Val(Sgnl)"=w300) -> ()  [unwired: 2 in, 2 out]
        n121 = property on="Overview Chart" class="WFChart (strict)"("XScale.ScaleFit"=w282) -> ()  [unwired: 2 in, 2 out]
        n122 = property on="Channel 0 Chart" class="WFChart (strict)"("XScale.ScaleFit"=w282) -> ()  [unwired: 2 in, 2 out]
        n123 = property on="Channel 1 Chart" class="WFChart (strict)"("XScale.ScaleFit"=w282) -> ()  [unwired: 2 in, 2 out]
        n124 = property on="Channel 2 Chart" class="WFChart (strict)"("XScale.ScaleFit"=w282) -> ()  [unwired: 2 in, 2 out]
        n125 = property on="Channel 3 Chart" class="WFChart (strict)"("XScale.ScaleFit"=w282) -> ()  [unwired: 2 in, 2 out]
      }
    }
    n126 = Get Notifier Status(notifier=w142, error in (no error)=w141) -> (current notification=w140:bool)  [unwired: 4 out]
    n127 = Or(x=w143, y=w140) -> (x .or. y?=w144:bool)
  }
  n128 = while {
    tunnel: w28 -> [w338]
    tunnel: w27 -> [w335]
    tunnel: [w337] -> w24
    tunnel: [w336] -> w23
    shift-right: [w323] -> _
    shift-left: Data_Producer_States."Default" -> [w316]
    shift-right: [w334] -> w17
    shift-left: _ -> [w332]
    shift-right: [w333] -> w16
    shift-left: _ -> [w331]
    tunnel: w9 -> [w328]
    tunnel: w8 -> [w327]
    shift-right: [w321] -> _
    shift-left: 0 -> [w322]
    tunnel: w2 -> [w318]
    tunnel: w1 -> [w317]
    stop <- w320 stop-if-true
    # "Producer Loop (Data)"
    n129 = Dequeue Element(queue=w328, timeout in ms (-1)=20, error in (no error)=w327) -> (element=w315:T1, timed out?=w326:bool)  [unwired: 2 out]
    n130 = Wait Until Next ms Multiple(millisecond multiple=u32 20) -> ()  [unwired: 1 out]
    n131 = Select(t=w316, s=w326, f=w315) -> (s? t:f=w325:T1)
    "Data Producer State" <- w325
    n132 = case shown="\"Read Data\"" w325 {
      tunnel: w338 -> [w352 w363 w372 w384]
      tunnel: [w350 w363 w372 w384] -> w337
      tunnel: [w349 w362 w371 w385] -> w336
      tunnel: w335 -> [w351 w362 w371 w385]
      tunnel: [w354 w361 w374 w386] -> w334
      tunnel: [w353 w360 w373 w387] -> w333
      tunnel: w332 -> [w356 w361 _ w386]
      tunnel: w331 -> [w355 w360 _ w387]
      tunnel: [FALSE FALSE FALSE TRUE] -> w329
      tunnel: [Data_Producer_States."Read Data" Data_Producer_States."Default" T14."Default" Data_Producer_States."Default"] -> w323
      tunnel: w322 -> [w345 _ _ _]
      tunnel: [w344 0 0 0] -> w321
      frame "Read Data" {
        n133 = call "Functional Global I32.vi"("Enum"=enum16{"Set Data", "Get Data"}."Get Data") -> ("Integer"=w341:i32)  [unwired: 10 in]
        n134 = Divide(x=w341, y=10) -> (x/y=w340:dbl)
        n135 = call-poly <vilib>:"DAQmxBase Read.vi"("task/channels in"=w356, "number of samples per channel"=w340, "timeout"=100.0, "error in"=w355) -> ("task out"=w354:refnum<k21>, "data"=w339:dbl[][], "error out"=w353:errorcluster)  [unwired: 9 in]
        n136 = Increment(x=w345) -> (x+1=w344:i32)
        "Read Data" <- w344
        n137 = Enqueue Element(queue=w352, element=w339, error in (no error)=w351) -> (queue out=w350:refnum<queue>, error out=w349:errorcluster)  [unwired: 1 in, 1 out]
      }
      frame "Default", Default {
      }
      frame "Set Sample Clock" {
        w364 = 10123 items=["Finite Samples"=10178, "Continuous Samples"=10123, "Hardware Timed Single Point"=12522] ("sample mode")
        n138 = property on="Sample Rate" class="DigNum (strict)"("DisabledEnum"=T7."Disabled and Grayed Out" ("Disabled")) -> ()  [unwired: 2 in, 2 out]
        n139 = call <vilib>:"DAQmxBase Create Task.vi"() -> ("task out"=w380:refnum<k21>, "error out"=w379:errorcluster)  [unwired: 14 in]
        n140 = call-poly <vilib>:"DAQmxBase Create Virtual Channel.vi"("task in"=w380, "physical channels"=tag "Dev1/ai0,Dev1/ai1,Dev1/ai2,Dev1/ai3", "error in"=w379) -> ("task out"=w377:refnum<k21>, "error out"=w378:errorcluster)  [unwired: 11 in]
        n141 = call-poly <vilib>:"DAQmxBase Timing.vi"("task/channels in"=w377, "sample mode"=w364, "rate"="Sample Rate", "error in"=w378) -> ("task out"=w376:refnum<k21>, "error out"=w375:errorcluster)  [unwired: 10 in]
        n142 = call "Functional Global I32.vi"("Enum"=enum16{"Set Data", "Get Data"}."Set Data", "Integer In"="Sample Rate") -> ()  [unwired: 9 in, 1 out]
        n143 = call <vilib>:"DAQmxBase Start Task.vi"("task/channels in"=w376, "error in"=w375) -> ("task out"=w374:refnum<k21>, "error out"=w373:errorcluster)  [unwired: 12 in]
      }
      frame "Exit" {
      }
    }
    n144 = Get Notifier Status(notifier=w318, error in (no error)=w317) -> (current notification=w319:bool)  [unwired: 4 out]
    n145 = Or(x=w329, y=w319) -> (x .or. y?=w320:bool)
  }
  n146 = Release Queue(queue=w26, error in (no error)=w25) -> ()  [unwired: 1 in, 3 out]
  n147 = Release Queue(queue=w24, error in (no error)=w23) -> (error out=w15:errorcluster)  [unwired: 1 in, 2 out]
  n148 = call <vilib>:"DAQmxBase Clear Task.vi"("task in"=w17, "error in"=w16) -> ("error out"=w14:errorcluster)  [unwired: 13 in]
  n149 = Merge Errors(w15, w14) -> (w13:errorcluster)
  n150 = call <vilib>:"Simple Error Handler.vi"("error in (no error)"=w13) -> ()  [unwired: 4 in, 5 out]
